vi "Get Session.vi"(8 "error in (no error)":errorcluster, 11 "WebDAV in":refnum<class "WebDAV.lvclass">) -> (0 "error out":errorcluster, 2 "session handle":T1, 3 "WebDAV out":refnum<class "WebDAV.lvclass">)   [LabVIEW 2016, in "RT Management.lvlib" / "WebDAV.lvclass"]
uses:
  WebDAV.lvclass
  <vilib>/WebDAVClient/Advanced/SessionHandle.ctl
  WebDAV.lvclass/WebDAV.ctl
  <vilib>/WebDAVClient/NI_WebDAV.lvlib
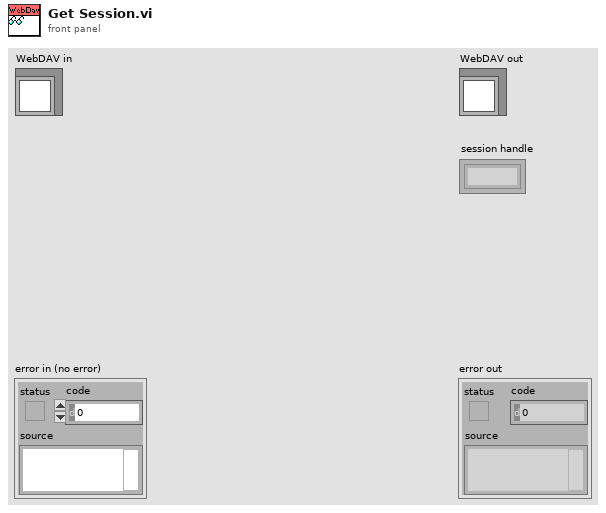
[diagram p1: front panel]
types:
  T1 = typedef "NI_WebDAV.lvlib/SessionHandle.ctl" = refnum<k1>
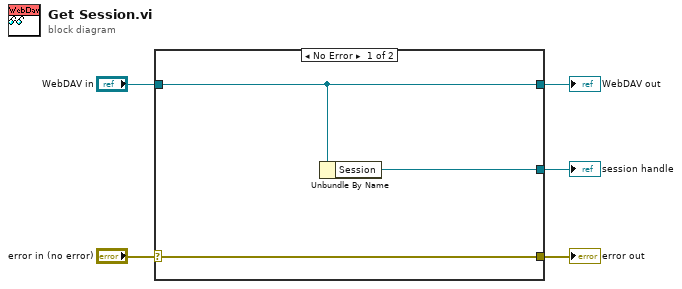
[diagram p0: block diagram]
diagram:
  n1 = case shown="No Error" "error in (no error)" {
    selector: "error in (no error)" -> [w8 w9]
    tunnel: [w8 w9] -> w4
    tunnel: [w7 w10] -> w2
    tunnel: "WebDAV in" -> [w7 w10]
    tunnel: [w6 _] -> w1
    frame No Error {
      n2 = Unbundle By Name(w7) -> ("Session"=w6:T1)
    }
    frame Error {
    }
  }
  "error out" <- w4
  "WebDAV out" <- w2
  "session handle" <- w1
